vi "SubVI_SpeedLimitMsgFW_Auto.vi"(11 "speed":string) -> (3 "Speed Limit":dbl)   [LabVIEW 2017]
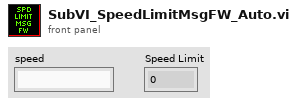
[diagram p1: front panel]
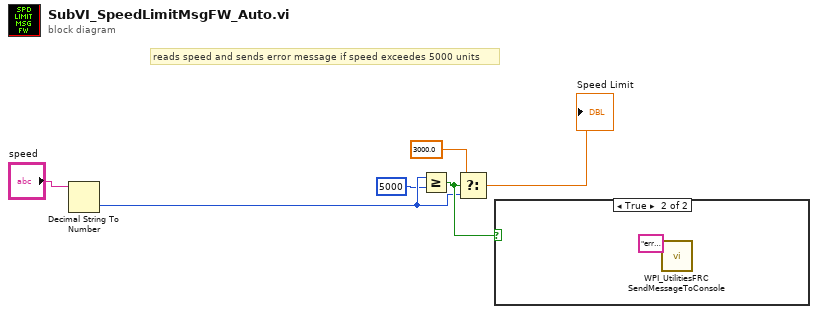
[diagram p0: block diagram]
diagram:
  # "reads speed and sends error message if speed exceedes 5000 units"
  n1 = Decimal String To Number(string="speed") -> (number=w4:i32)  [unwired: 2 in, 1 out]
  n2 = Greater Or Equal?(x=w4, y=5000) -> (x >= y?=w6:bool)
  n3 = Select(t=3000.0, s=w6, f=w4) -> (s? t:f=→"Speed Limit":dbl)
  n4 = case shown="True" w6 {
    frame False {
    }
    frame True {
      n5 = call <vilib>:"WPI_UtilitiesFRC SendMessageToConsole.vi"("Message"="error your speed has exceeded 5000 and is being blocked by autonomous independent VI") -> ()  [unwired: 14 in, 1 out]
    }
  }
